vi "Obtain Request Events.vi"(8 "error in (no error)":errorcluster, 10 "Create New?":bool) -> (0 "error out":errorcluster, 2 "GenNet-Server Request Events":T1)   [LabVIEW 2022 SP3, in "GenNet-Server.lvlib"]
doc: "This VI Obtains/Creates the Requests events that will be used for other modules to communicate with the module that owns this VI. These Requests events will be accessed only via Public API methods for this module.\n\n<b>NOTE</b>: The contents of this VI are automatically generated and modified by the <b>Tools > Delacor > DQMH</b> utilities. Consider using those utilities instead of making your own modifications to this VI.\n____\nHAMPEL SOFTWARE ENGINEERING v3.8.0 (2023-12-18 14:41)"
uses:
  GenNet-Server.lvlib
  Request Events--cluster.ctl
  Stop Argument--cluster.ctl
  Show Panel Argument--cluster.ctl
  Hide Panel Argument--cluster.ctl
  Show Diagram Argument--cluster.ctl
  Get Module Execution Status Argument--cluster.ctl
  Forward Generic Broadcasts to Network Argument--cluster.ctl
  UDP Broadcasting/Generic Broadcasts.ctl
  hse-dqmh/Dynamic Requesters/Singleton/Status Updated Argument--cluster.ctl
  hse-dqmh/Dynamic Requesters/Singleton/Error Reported Argument--cluster.ctl
  hse-dqmh/Dynamic Requesters/Singleton/Get Module Execution Status Argument--cluster.ctl
  hse-dqmh/Dynamic Requesters/Singleton/Stop Argument--cluster.ctl
  hse-dqmh/Controls/System Message Argument--cluster.ctl
  hse-dqmh/Controls/System Message Source.ctl
  UDP Broadcasting/Network Broadcast Params.ctl
  hse-gennet.lvlib
  hse-dqmh/hse-dqmh.lvlib
  hse-dqmh/hse-dqmh-dynamicrequesters.lvlib
panel:
  # "NOTE: The contents of this VI are automatically generated and modified by the Tools > Delacor > DQMH utilities. Consider using those utilities instead of making your own modifications to this VI."
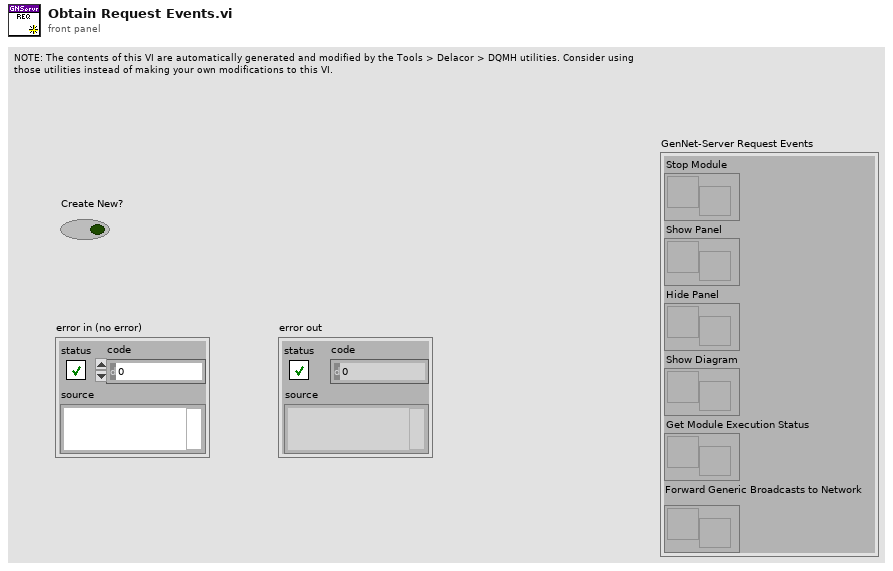
[diagram p1: front panel]
types:
  T1 = typedef "GenNet-Server.lvlib/Request Events--cluster.ctl" = cluster{"Stop Module":refnum<user-event>, "Show Panel":refnum<user-event>, "Hide Panel":refnum<user-event>, "Show Diagram":refnum<user-event>, "Get Module Execution Status":refnum<user-event>, "Forward Generic Broadcasts to Network":refnum<user-event>}
  T2 = typedef "GenNet-Server.lvlib/Forward Generic Broadcasts to Network Argument--cluster.ctl" = cluster{"Module ID":i32, "Generic Broadcast Events":T3, "Network Broadcast Params":T4}
  T3 = typedef "hse-gennet.lvlib/Generic Broadcasts.ctl" = cluster{"Status Updated":refnum<user-event>, "Error Reported":refnum<user-event>, "Update Module Execution Status":refnum<user-event>, "Module Did Stop":refnum<user-event>, "System Message":refnum<user-event>}
  T4 = typedef "hse-gennet.lvlib/Network Broadcast Params.ctl" = cluster{"Server (Sender) Port":u16, "Client (Receiver) Port":u16, "Multicast Address":string, "Local IP Address":string, "Max Rx Byte Size":i32}
  T5 = typedef "GenNet-Server.lvlib/Get Module Execution Status Argument--cluster.ctl" = cluster{"Module ID":i32, "Running?":bool}
  T6 = typedef "GenNet-Server.lvlib/Show Diagram Argument--cluster.ctl" = cluster{"Module ID":i32, "Debug?":bool}
  T7 = typedef "GenNet-Server.lvlib/Show Panel Argument--cluster.ctl" = cluster{"Show Panel?":bool, "Module ID":i32}
  T8 = typedef "GenNet-Server.lvlib/Hide Panel Argument--cluster.ctl" = cluster{"Hide Panel?":bool, "Module ID":i32}
  T9 = typedef "GenNet-Server.lvlib/Stop Argument--cluster.ctl" = cluster{"Origin":string, "Module ID":i32, "Exit via Stop Module Req?":bool, "Wait for Module to stop?":bool}
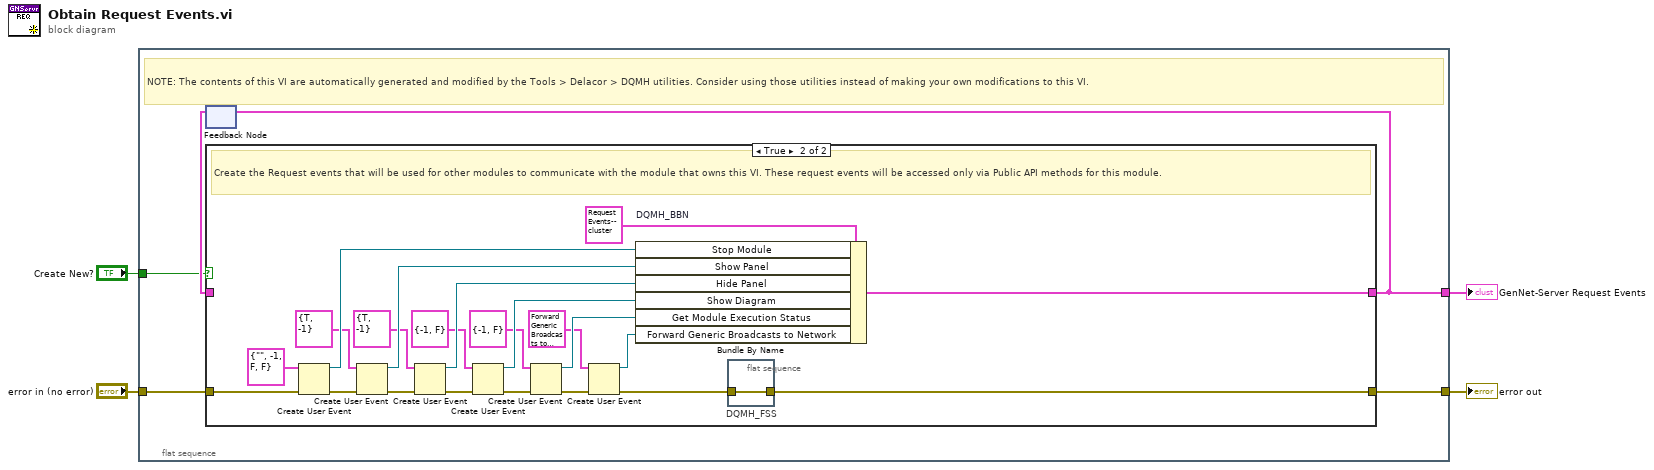
[diagram p0: block diagram]
diagram:
  n1 = flat-sequence {
    tunnel: [w9] -> w4
    tunnel: "error in (no error)" -> [w8]
    tunnel: [w6] -> w2
    tunnel: "Create New?" -> [w5]
    frame #0 {
      # "NOTE: The contents of this VI are automatically generated and modified by the Tools > Delacor > DQMH utilities. Consider using those utilities instead of making your own modifications to this VI."
      n2 = feedback #1() -> (w7:T1)  [unwired: 1 in]
      n3 = case shown="True" w5 {
        tunnel: [w10 w21] -> w9
        tunnel: w8 -> [w10 w33]
        tunnel: [w11 w30] -> w6
        tunnel: w7 -> [w11 _]
        frame False {
        }
        frame True {
          # "Create the Request events that will be used for other modules to communicate with the module that owns this VI. These request events will be accessed only via Public API methods for this module."
          n4 = Create User Event(user event datatype=T9 {"Origin"="", "Module ID"=-1, "Exit via Stop Module Req?"=FALSE, "Wait for Module to stop?"=FALSE} ("Stop Argument"), error in=w33) -> (user event=w31:refnum<user-event>, error out=w28:errorcluster)
          n5 = Create User Event(user event datatype=T7 {"Show Panel?"=TRUE, "Module ID"=-1} ("Show Panel Argument"), error in=w28) -> (user event=w27:refnum<user-event>, error out=w25:errorcluster)
          n6 = Create User Event(user event datatype=T8 {"Hide Panel?"=TRUE, "Module ID"=-1} ("Hide Panel"), error in=w25) -> (user event=w24:refnum<user-event>, error out=w23:errorcluster)
          n7 = Create User Event(user event datatype=T6 {"Module ID"=-1, "Debug?"=FALSE} ("Show Diagram Argument"), error in=w23) -> (user event=w19:refnum<user-event>, error out=w20:errorcluster)
          n8 = Create User Event(user event datatype=T5 {"Module ID"=-1, "Running?"=FALSE} ("Get Module Execution Status Argument"), error in=w20) -> (user event=w16:refnum<user-event>, error out=w17:errorcluster)
          n9 = Create User Event(user event datatype=T2 {"Module ID"=-1, "Generic Broadcast Events"={"Status Updated"=refnum, "Error Reported"=refnum, "Update Module Execution Status"=refnum, "Module Did Stop"=refnum, "System Message"=refnum}, "Network Broadcast Params"={"Server (Sender) Port"=0, "Client (Receiver) Port"=0, "Multicast Address"="", "Local IP Address"="", "Max Rx Byte Size"=0}} ("Forward Generic Broadcasts to Network Argument"), error in=w17) -> (user event=w13:refnum<user-event>, error out=w14:errorcluster)
          n10 = Bundle By Name "DQMH_BBN"(cluster=T1 {"Stop Module"=refnum, "Show Panel"=refnum, "Hide Panel"=refnum, "Show Diagram"=refnum, "Get Module Execution Status"=refnum, "Forward Generic Broadcasts to Network"=refnum} ("output cluster"), "Stop Module"=w31, "Show Panel"=w27, "Hide Panel"=w24, "Show Diagram"=w19, "Get Module Execution Status"=w16, "Forward Generic Broadcasts to Network"=w13) -> (w30:T1)
          n11 = flat-sequence "DQMH_FSS" {
            tunnel: w14 -> [w34]
            tunnel: [w34] -> w21
            frame #0 {
            }
          }
        }
      }
      n12 = feedback-in #1(w6) -> ()
    }
  }
  "GenNet-Server Request Events" <- w2
  "error out" <- w4
